vi "Detector Control.vi"(9 "control_detector_reading":cluster{"x":i16, "y":i16, "sum":u16}, 11 "control_request":string) -> (2 "indicator_detector_reading":cluster{"x":i16, "y":i16, "sum":u16}, 3 "indicator_detector_status":bool)   [LabVIEW 2020]
uses:
  <vilib>/Utility/file.llb/Read Delimited Spreadsheet (string).vi
  Dependencies/Thorlabs/Thorlabs.MotionControl.KCube.PositionAligner.dll
panel:
  out "error out 2":errorcluster
  out "error out":errorcluster
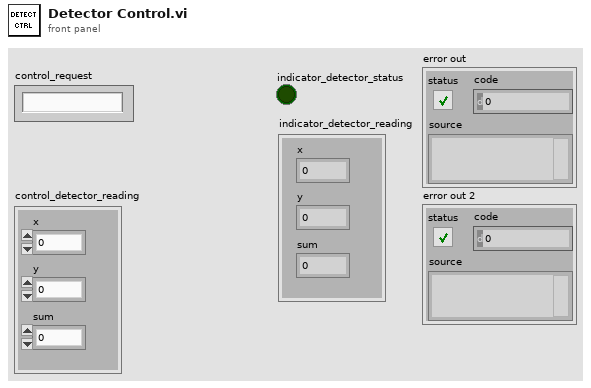
[diagram p1: front panel]
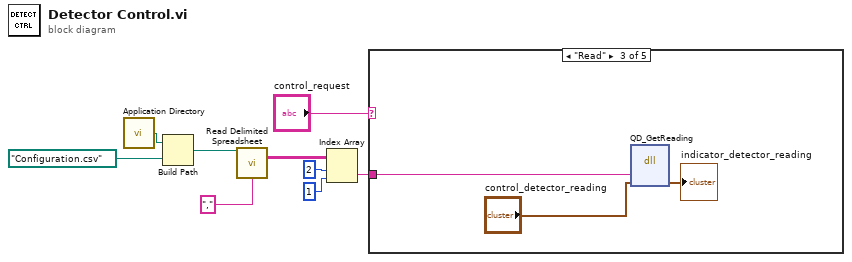
[diagram p0: block diagram]
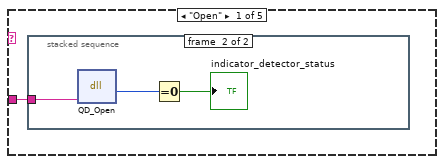
[diagram p2: hidden frame]
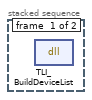
[diagram p3: hidden frame]
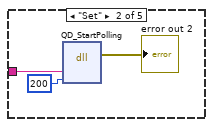
[diagram p4: hidden frame]
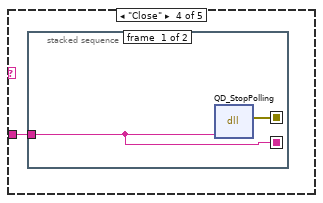
[diagram p5: hidden frame]
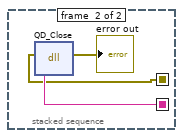
[diagram p6: hidden frame]
diagram:
  n1 = call <vilib>:"Application Directory.vi"() -> ("Application Directory"=w5:path)
  n2 = Build Path(base path=w5, name or relative path=path "Configuration.csv" ("file path (dialog if empty)")) -> (appended path=w4:path)
  n3 = call-poly <vilib>:"Read Delimited Spreadsheet.vi"("file path (dialog if empty)"=w4, "delimiter (\\t)"="," ("delimiter (\\t)")) -> ("all rows"=w2:string[][])  [unwired: 8 in, 5 out]
  n4 = Index Array(array=w2, index (row)=2, index (col)=1 ("disabled index (col)")) -> (element=w1:string)
  n5 = case shown="\"Read\"" "control_request" {
    tunnel: w1 -> [w10 w14 w17 w20 _]
    frame "Open" {
      n6 = stacked-sequence {
        tunnel: w10 -> [_ w11]
        frame #0 {
          n7 = dll-call lib="C:/Users/Klenerman/Desktop/Control Software/Dependencies/Thorlabs/Thorlabs.MotionControl.KCube.PositionAligner.dll" fn="TLI_BuildDeviceList"() -> ()  [unwired: 4 in, 2 out]
        }
        frame #1 {
          n8 = dll-call lib="C:/Users/Klenerman/Desktop/Control Software/Dependencies/Thorlabs/Thorlabs.MotionControl.KCube.PositionAligner.dll" fn="QD_Open"("serialNo"=w11) -> ("return type"=w13:i16)  [unwired: 4 in, 2 out]
          n9 = Equal To 0?(x=w13) -> (x = 0?=→"indicator_detector_status":bool)
        }
      }
    }
    frame "Set" {
      n10 = dll-call lib="C:/Users/Klenerman/Desktop/Control Software/Dependencies/Thorlabs/Thorlabs.MotionControl.KCube.PositionAligner.dll" fn="QD_StartPolling"("serialNo"=w14, "milliseconds"=i16 200) -> (error out=→"error out 2":errorcluster)  [unwired: 6 in, 1 out]
    }
    frame "Read" {
      n11 = dll-call lib="C:/Users/Klenerman/Desktop/Control Software/Dependencies/Thorlabs/Thorlabs.MotionControl.KCube.PositionAligner.dll" fn="QD_GetReading"("serialNo"=w17, "indicator_detector_reading"="control_detector_reading") -> ("indicator_detector_reading"=→"indicator_detector_reading":cluster{"x":i16, "y":i16, "sum":u16})  [unwired: 5 in, 2 out]
    }
    frame "Close" {
      n12 = stacked-sequence {
        seq-local: [w21 _] -> [_ w25]
        seq-local: [w22 _] -> [_ w24]
        tunnel: w20 -> [w21 _]
        frame #0 {
          n13 = dll-call lib="C:/Users/Klenerman/Desktop/Control Software/Dependencies/Thorlabs/Thorlabs.MotionControl.KCube.PositionAligner.dll" fn="QD_StopPolling"("serialNo"=w21) -> (error out=w22:errorcluster)  [unwired: 5 in, 1 out]
        }
        frame #1 {
          n14 = dll-call lib="C:/Users/Klenerman/Desktop/Control Software/Dependencies/Thorlabs/Thorlabs.MotionControl.KCube.PositionAligner.dll" fn="QD_Close"(error in=w24, "serialNo"=w25) -> (error out=→"error out":errorcluster)  [unwired: 4 in, 1 out]
        }
      }
    }
    frame "Default", Default {
    }
  }
